vi "Close.vi"(8 "error in (no error)":errorcluster, 11 "_ConfigClass_INI_IN":refnum<class "_ConfigClass_INI.lvclass">) -> (0 "error out":errorcluster, 3 "_ConfigClass_INI_OUT":refnum<class "_ConfigClass_INI.lvclass">)   [LabVIEW 2019, in "_ConfigClass_INI.lvlib" / "_ConfigClass_INI.lvclass"]
uses:
  _ConfigClass_INI.lvclass
  <vilib>/Utility/config.llb/NI_LVConfig.lvlib
  <vilib>/Utility/config.llb/Config Data RefNum.ctl
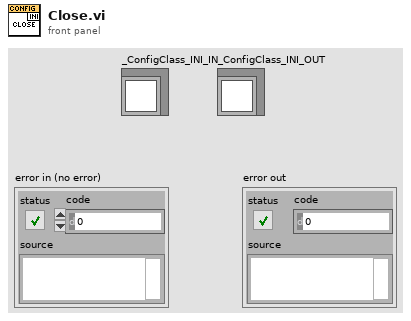
[diagram p1: front panel]
types:
  T1 = typedef "NI_LVConfig.lvlib/Config Data RefNum.ctl" = refnum<k1>
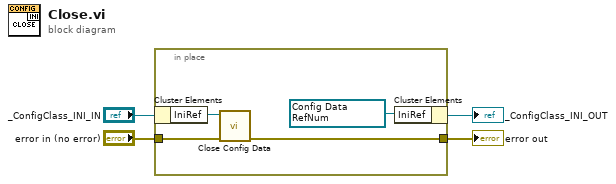
[diagram p0: block diagram]
diagram:
  n1 = in-place {
    in-place-border: "error in (no error)" -> [w8]
    in-place-border: [w6] -> w1
    w5 = T1 refnum items=["config data"] ("IniRef")
    n2 = in-place-cluster #1("_ConfigClass_INI_IN") -> ("IniRef"=w7:T1)
    n3 = call <vilib>:"Close Config Data.vi"("error in (no error)"=w8, "refnum"=w7) -> ("error out"=w6:errorcluster)  [unwired: 8 in, 1 out]
    n4 = in-place-cluster #1("IniRef"=w5) -> (→"_ConfigClass_INI_OUT":refnum<class "_ConfigClass_INI.lvclass">)
  }
  "error out" <- w1
